vi "File_Save png Glyph List.vi"(8 "error in (no error)":errorcluster, 11 "Glyph list":T1=[{"Install"=FALSE, "Current"=bytes[272], "Icon Library"=bytes[272], "Subfolder"="", "Name"=""}]) -> (0 "error out":errorcluster)   [LabVIEW 2021]
uses:
  TypeDefs/Array_Glyph List.ctl
  TypeDefs/Cluster_Glyph Data.ctl
  vi.lib/LabVIEW Icon API/lv_icon/Controls/Pathes.ctl
  vi.lib/LabVIEW Icon API/lv_icon/lv_icon.lvlib
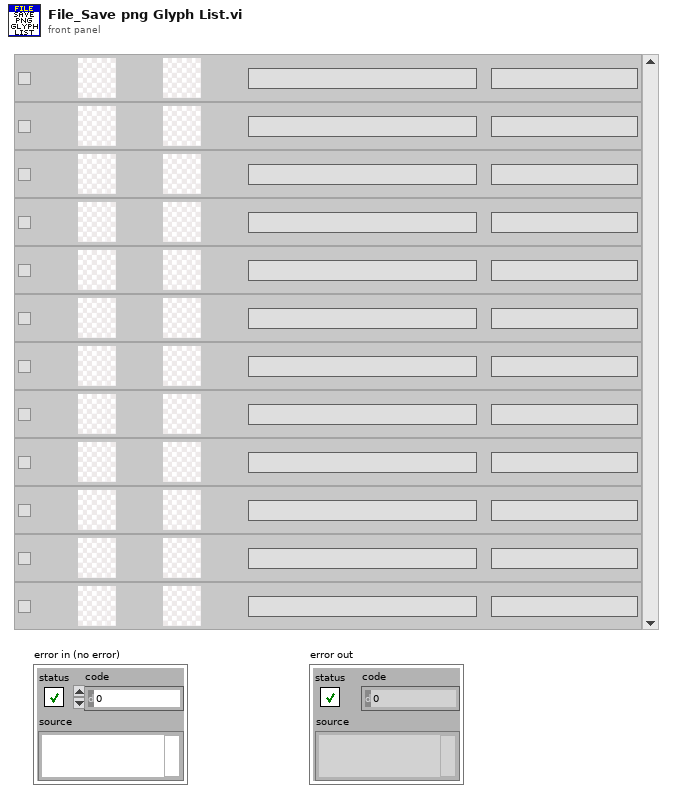
[diagram p1: front panel]
types:
  T1 = typedef "Array_Glyph List.ctl" = T2[]
  T2 = typedef "Cluster_Glyph Data.ctl" = cluster{"Install":bool, "Current":picture, "Icon Library":picture, "Subfolder":string, "Name":string}
  T3 = typedef "Pathes.ctl" = enum16{"Root Path", "Icon Templates", "Icon Templates VI", "Icon Templates Lib", "Glyphs"}
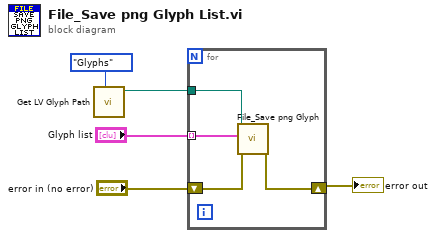
[diagram p0: block diagram]
diagram:
  n1 = call "Get LV Glyph Path.vi"("Path"=Pathes."Glyphs") -> ("Requested Path"=w3:path)  [unwired: 2 in, 8 out]
  n2 = for {
    tunnel: "Glyph list" -> [w9] mode=indexing
    tunnel: w3 -> [w8]
    shift-right: [w6] -> w1
    shift-left: "error in (no error)" -> [w7]
    n3 = call "File_Save png Glyph.vi"("Error"=w7, "Glyph Data"=w9, "Starting Folder"=w8) -> ("Error Out"=w6:errorcluster)  [unwired: 8 in]
  }
  "error out" <- w1
